vi "configure operation.vi"(7 "owner ID":refnum<class "Profibus Module configuration.lvclass">, 8 "error in":errorcluster, 10 "line item in":T1, 11 "engine configuration in":refnum<class "engine configuration.lvclass">) -> (0 "error out":errorcluster, 1 "success":bool, 2 "line item out":T1, 5 "changed":bool)   [LabVIEW 2013, in "Profibus Module editor node.lvclass"]
uses:
  Profibus Module editor node.lvclass
  permissions.ctl
  table line.ctl
  channel/Profibus channel.lvclass
  <vilib>/NI/Module Execution Interface/Engine Configuration/engine configuration.lvclass
  configuration/Profibus Module configuration.lvclass
  <vilib>/NI/Configuration Framework/serializable configuration/NISE_CEF_serializable configuration.lvclass/NISE_CEF_serializable configuration.ctl
  <vilib>/NI/Configuration Framework/serializable configuration/NISE_CEF_serializable configuration.lvclass
  <vilib>/NI/Tag Bus Module Framework/channel/TBM channel.lvclass/TBM channel.ctl
  <vilib>/NI/Tag Bus/tag/tag descriptor.lvclass/tag descriptor.ctl
  channel/Profibus channel.lvclass/Profibus channel.ctl
  <vilib>/NI/Tag Bus/tag/Data Type.ctl
  <vilib>/NI/Configuration Framework/serializable configuration/Read UID.vi
  <vilib>/NI/Tag Bus Module Framework/channel/Read channel classification.vi
  <vilib>/NI/Tag Bus/tag/read data type.vi
  channel/Read slave.vi
  channel/Read byte.vi
  channel/Read bit.vi
  <vilib>/NI/Tag Bus/tag/write tag name.vi
  <vilib>/NI/Tag Bus/tag/write data type.vi
  <vilib>/NI/Tag Bus Module Framework/channel/Write channel classification.vi
  channel/Write slave.vi
  channel/Write byte.vi
  channel/Write bit.vi
  <vilib>/NI/Tag Bus/tag/tag descriptor.lvclass
panel:
  in  "Linked Tag":i32(listbox)
  in  "Type":i32(listbox)
  in  "bit":i32
  in  "byte":i32
  in  "slave":i8
  in  "Channel Name":string
  in  "cancel":bool
  in  "ok":bool
  in  "Access Type":T2
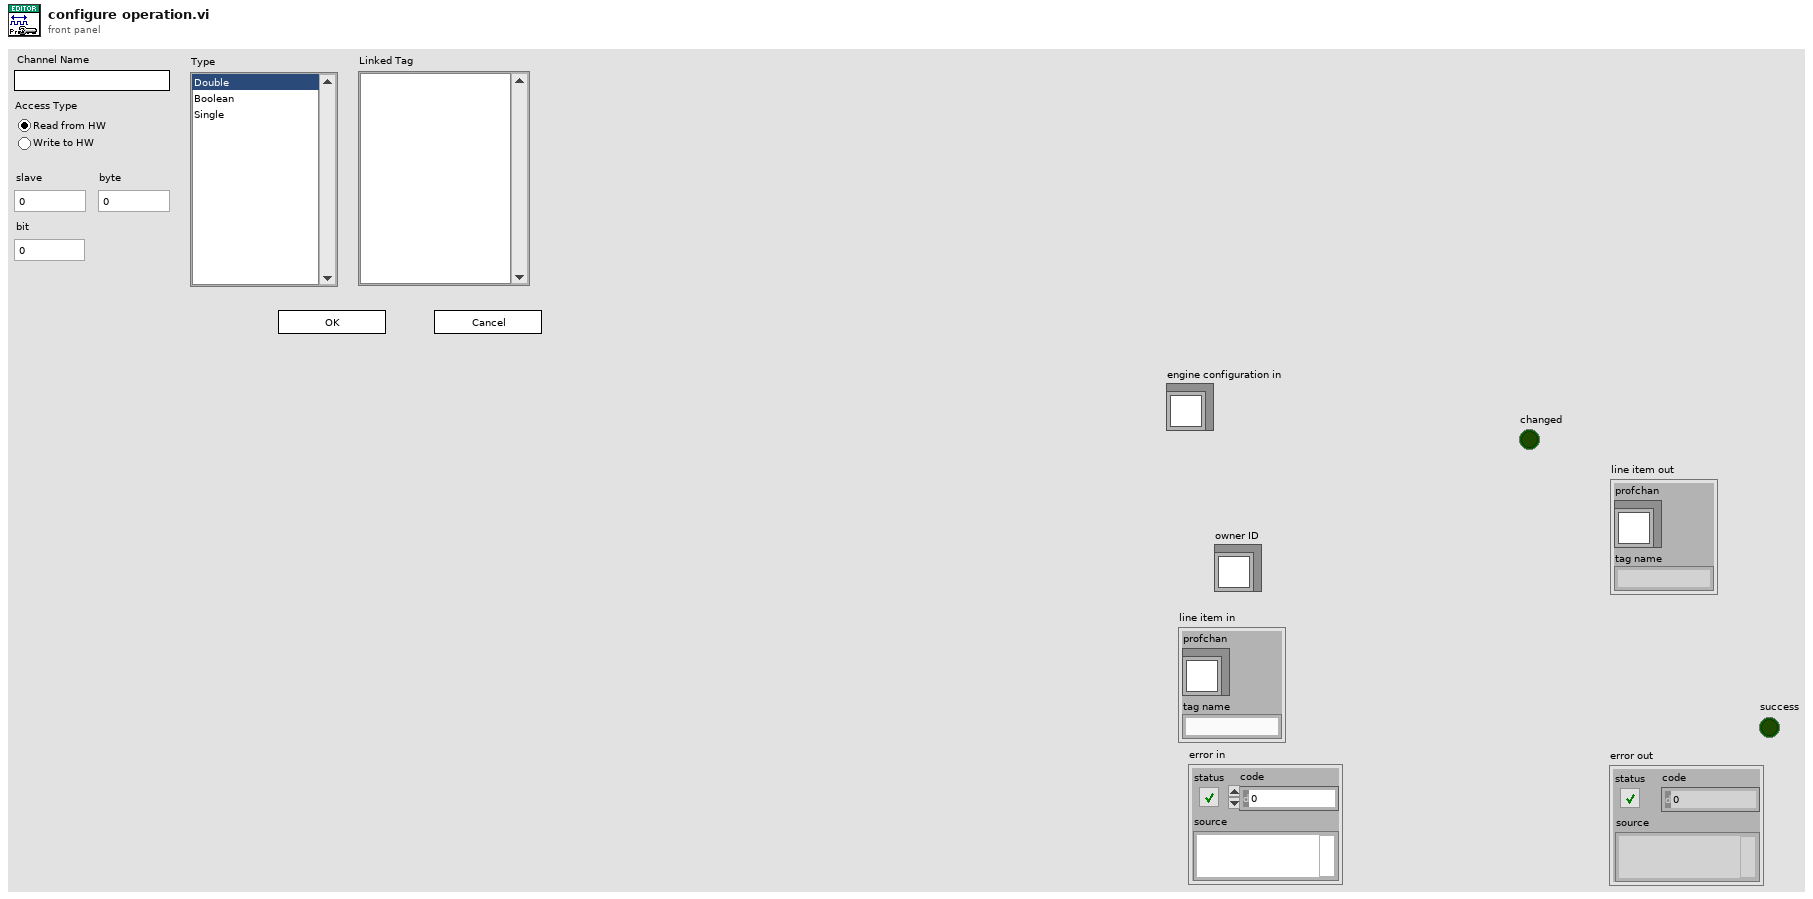
[diagram p1: front panel]
types:
  T1 = typedef "Profibus Module editor node.lvclass/table line.ctl" = cluster{"profchan":refnum<class "Profibus channel.lvclass">, "tag name":string}
  T2 = typedef "Profibus Module editor node.lvclass/permissions.ctl" = enum32{"Read from HW", "Write to HW"}
  T3 = enum32{"Invalid", "Standard", "Closed", "Hidden", "Minimized", "Maximized"}
  T4 = enum32{"Invalid", "Default", "Floating", "Floating/Auto-Hide", "Modal"}
  T5 = enum8{"Enabled", "Disabled", "Disabled and Grayed Out"}
  T6 = typedef "tag bus.lvlib/tag descriptor.lvclass/Data Type.ctl" = enum16{"Double", "Single", "I64", "I32", "I16", "I8", "U64", "U32", "U16", "U8", "Boolean", "String", "Array of Double", "Array of Single", "Array of I64", "Array of I32", "Array of I16", "Array of I8", "Array of U64", "Array of U32", "Array of U16", "Array of U8", "Array of Boolean", "Array of String"}
  T7 = enum32{"invalid app kind", "Development System", "Run Time System", "Student Edition", "Embedded LabVIEW", "Evaluation", "Custom"}
  T8 = typedef "TBM channel.lvclass/channel classification.ctl" = enum16{"input data", "output data", "processing parameter", "processing result"}
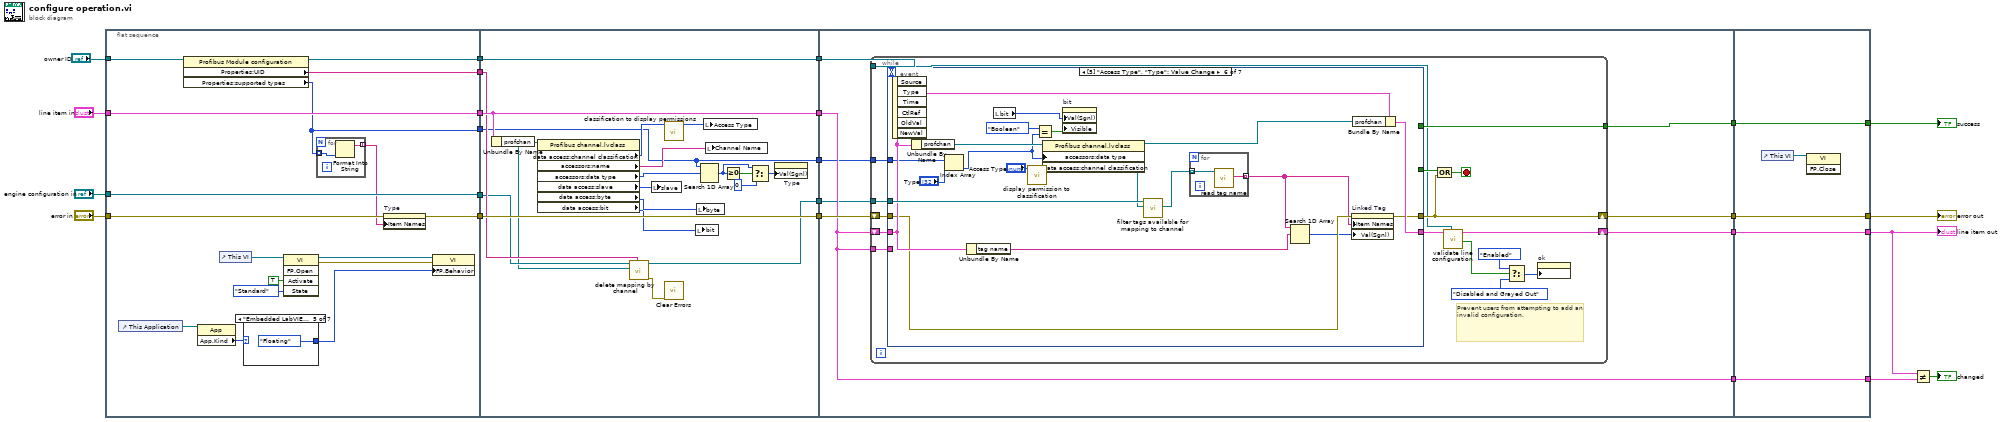
[diagram p0: block diagram]
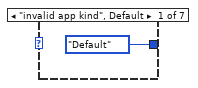
[diagram p2: hidden frame]
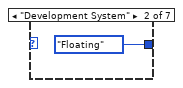
[diagram p3: hidden frame]
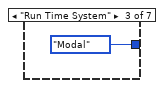
[diagram p4: hidden frame]
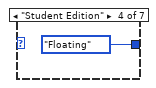
[diagram p5: hidden frame]
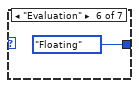
[diagram p6: hidden frame]
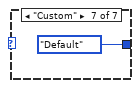
[diagram p7: hidden frame]
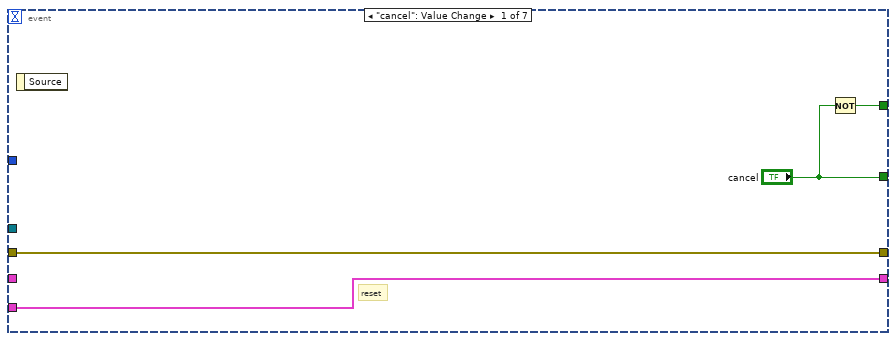
[diagram p8: hidden frame]
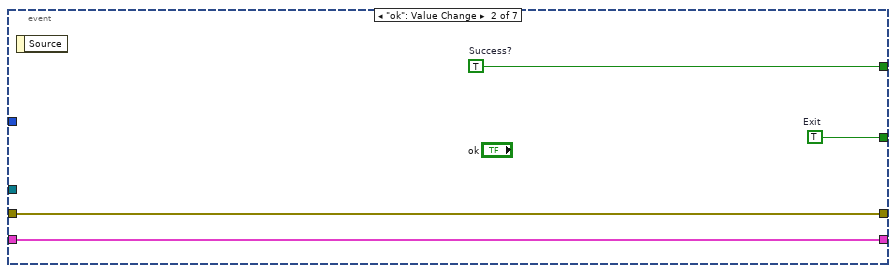
[diagram p9: hidden frame]
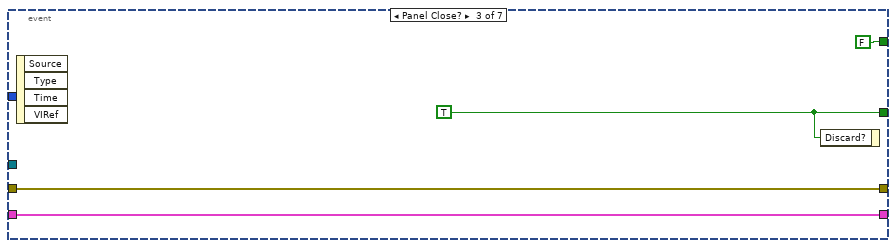
[diagram p10: hidden frame]
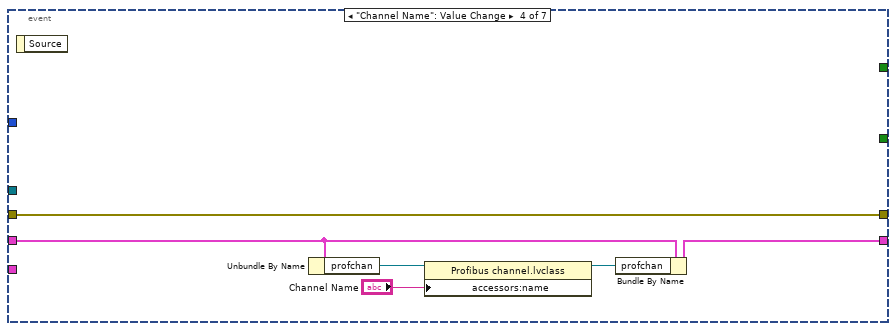
[diagram p11: hidden frame]
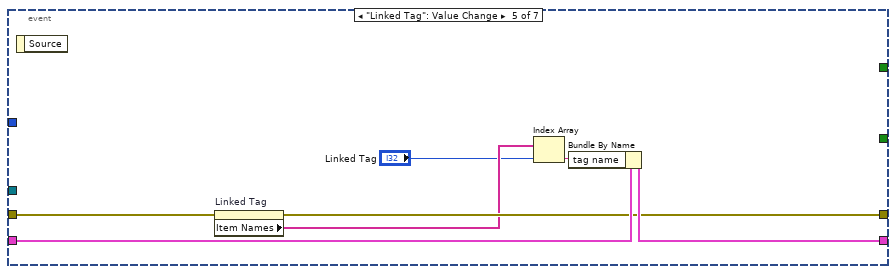
[diagram p12: hidden frame]
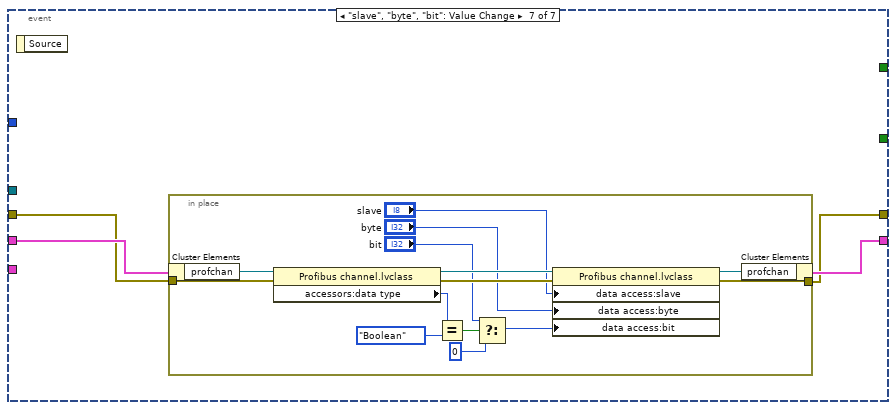
[diagram p13: hidden frame]
diagram:
  n1 = flat-sequence {
    tunnel: "line item in" -> [w41]
    tunnel: "error in" -> [w28]
    tunnel: [w27] -> w13
    tunnel: [w41] -> w11
    tunnel: [w30] -> w8
    tunnel: "owner ID" -> [w32]
    tunnel: [w31] -> w6
    tunnel: "engine configuration in" -> [w31]
    tunnel: [w29] -> w3
    tunnel: [w25] -> w2
    tunnel: w13 -> [w70]
    tunnel: [w70] -> w12
    tunnel: w11 -> [w66]
    tunnel: [w66] -> w10
    tunnel: [w62] -> w9
    tunnel: w8 -> [w62]
    tunnel: w6 -> [w59]
    tunnel: [w61] -> w4
    tunnel: w3 -> [w60]
    tunnel: w2 -> [w52]
    tunnel: [w52] -> w1
    tunnel: [w77] -> w17
    tunnel: [w76] -> w16
    tunnel: [w75] -> w15
    tunnel: [w74] -> w14
    tunnel: w12 -> [w78]
    tunnel: w10 -> [w74]
    tunnel: w9 -> [w73]
    tunnel: w4 -> [w72]
    tunnel: w1 -> [w71]
    tunnel: [w160] -> w18
    tunnel: [w161] -> w21
    tunnel: [w162] -> w22
    tunnel: [w163] -> w23
    tunnel: w17 -> [w163]
    tunnel: w16 -> [w162]
    tunnel: w15 -> [w161]
    tunnel: w14 -> [w160]
    frame #0 {
      n2 = control-ref of="This Application"() -> (w35:refnum<vi>)
      n3 = property class="Profibus Module configuration"(reference=w32) -> (reference out=w30:refnum<class "Profibus Module configuration.lvclass">, "Properties:UID"=w29:string, "Properties:supported types"=w25:T6[])  [unwired: 1 in, 1 out]
      n4 = property class="App"(reference=w35) -> ("App.Kind"=w34:T7)  [unwired: 1 in, 2 out]
      n5 = control-ref of="This VI"() -> (w36:refnum<vi>)
      n6 = case shown="\"Embedded LabVIEW\"" w34 {
        tunnel: [T4."Default" ("Front Panel Window:Behavior") T4."Floating" ("Front Panel Window:Behavior") T4."Modal" ("Front Panel Window:Behavior") T4."Floating" ("Front Panel Window:Behavior") T4."Floating" ("Front Panel Window:Behavior") T4."Floating" ("Front Panel Window:Behavior") T4."Default" ("Front Panel Window:Behavior")] -> w33
        frame "invalid app kind", Default {
        }
        frame "Development System" {
        }
        frame "Run Time System" {
        }
        frame "Student Edition" {
        }
        frame "Embedded LabVIEW" {
        }
        frame "Evaluation" {
        }
        frame "Custom" {
        }
      }
      n7 = invoke class="VI" method="FP.Open"(reference=w36, "Activate"=TRUE ("Activate?"), "State"=T3."Standard") -> (reference out=w39:refnum<vi>, error out=w40:errorcluster)  [unwired: 2 in, 3 out]
      n8 = for {
        tunnel: w25 -> [w43] mode=indexing
        tunnel: [w42] -> w26 mode=indexing
        n9 = Format Into String(w43) -> (resulting string=w42:string)  [unwired: 3 in, 1 out]
      }
      n10 = property on="Type" class="LstBox (strict)"(error in=w28, "Item Names"=w26) -> (error out=w27:errorcluster)  [unwired: 1 in, 1 out]
      n11 = property class="VI"(reference=w39, error in=w40, "FP.Behavior"=w33) -> ()  [unwired: 2 out]
    }
    frame #1 {
      n12 = Unbundle By Name(w66) -> ("profchan"=w58:refnum<class "Profibus channel.lvclass">)
      n13 = property class="Profibus channel.lvclass"(reference=w58) -> ("data access:channel classification"=w69:T8, "accessors:name"=w68:string, "accessors:data type"=w56:T6, "data access:slave"=w63:i8, "data access:byte"=w65:i32, "data access:bit"=w64:i32)  [unwired: 1 in, 2 out]
      n14 = call <vilib>:"delete mapping by channel.vi"("owner ID"=w60, "channel"=w58, "engine configuration in"=w59) -> ("error out"=w57:errorcluster, "engine configuration out"=w61:refnum<class "engine configuration.lvclass">)  [unwired: 7 in]
      n15 = local write "slave"(w63) -> ()
      n16 = call "classification to display permissions.vi"("channel classification"=w69) -> ("permissions"=w67:T2)  [unwired: 10 in]
      n17 = call <vilib>:"Clear Errors.vi"("error in (no error)"=w57) -> ()  [unwired: 6 in, 1 out]
      n18 = local write "bit"(w64) -> ()
      n19 = local write "byte"(w65) -> ()
      n20 = Search 1D Array(1D array=w52, element=w56) -> (index of element=w54:i32)  [unwired: 1 in]
      n21 = local write "Access Type"(w67) -> ()
      n22 = local write "Channel Name"(w68) -> ()
      n23 = Greater Or Equal To 0?(x=w54) -> (x >= 0?=w55:bool)
      n24 = Select(t=w54, s=w55, f=0) -> (s? t:f=w51:i32)
      n25 = property on="Type" class="LstBox (strict)"("Val(Sgnl)"=w51) -> ()  [unwired: 2 in, 2 out]
    }
    frame #2 {
      n26 = while {
        shift-right: [w86] -> w76
        shift-left: w78 -> [w81]
        tunnel: [w93] -> w77
        shift-right: [w87] -> w75
        shift-left: w74 -> [w90]
        tunnel: w74 -> [w89]
        tunnel: w73 -> [w80]
        tunnel: w71 -> [w79]
        tunnel: w72 -> [w94]
        stop <- w91 stop-if-true
        # "Prevent users from attempting to add an invalid configuration."
        n27 = event shown="[5] \"Access Type\", \"Type\": Value Change" {
          selector: _ -> [_ _ _ _ _ _ _]
          dyn-events: _ -> [_ _ _ _ _ _ _]
          timeout: _ -> [_ _ _ _ _ _ _]
          tunnel: w94 -> [_ _ _ _ _ w136 _]
          tunnel: w81 -> [w98 w102 w106 w112 w116 w123 w141]
          tunnel: [w98 w102 w106 w112 w115 w124 w142] -> w86
          tunnel: [w97 w99 FALSE _ _ _ _] -> w93
          tunnel: ["cancel" w100 w104 _ _ _ _] -> w92
          tunnel: w90 -> [_ w101 w103 w110 w119 w134 w144]
          tunnel: [w95 w101 w103 w111 w118 w128 w143] -> w88
          tunnel: w89 -> [w95 _ _ _ _ _ _]
          tunnel: w79 -> [_ _ _ _ _ w127 _]
          event "cancel": Value Change {
            # "reset"
            n28 = event-data() -> ()  [unwired: 1 in, 1 out]
            n29 = Not(x="cancel") -> (.not. x?=w97:bool)
          }
          event "ok": Value Change {
            w99 = TRUE  # Success?
            w100 = TRUE  # Exit
            n30 = event-data() -> ()  [unwired: 1 in, 1 out]
          }
          event Panel Close? {
            w104 = TRUE ("cancel")
            n31 = event-data() -> ()  [unwired: 1 in, 4 out]
            n32 = event-data("Discard?"=w104) -> ()  [unwired: 1 in, 1 out]
          }
          event "Channel Name": Value Change {
            n33 = event-data() -> ()  [unwired: 1 in, 1 out]
            n34 = Unbundle By Name(w110) -> ("profchan"=w109:refnum<class "Profibus channel.lvclass">)
            n35 = property class="Profibus channel.lvclass"(reference=w109, "accessors:name"="Channel Name") -> (reference out=w108:refnum<class "Profibus channel.lvclass">)  [unwired: 1 in, 1 out]
            n36 = Bundle By Name(cluster=w110, "profchan"=w108) -> (w111:T1)
          }
          event "Linked Tag": Value Change {
            n37 = event-data() -> ()  [unwired: 1 in, 1 out]
            n38 = property on="Linked Tag" class="LstBox (strict)"(error in=w116) -> (error out=w115:errorcluster, "Item Names"=w114:string[])  [unwired: 1 in, 1 out]
            n39 = Index Array(array=w114, index="Linked Tag") -> (element=w117:string)
            n40 = Bundle By Name(cluster=w119, "tag name"=w117) -> (w118:T1)
          }
          event "Type": Value Change {
            n41 = event-data() -> ()  [unwired: 1 in, 6 out]
            n42 = Unbundle By Name(w134) -> ("profchan"=w129:refnum<class "Profibus channel.lvclass">)
            n43 = Index Array(array=w127, index="Type") -> (element=w125:T6)
            n44 = Unbundle By Name(w134) -> ("tag name"=w121:string)
            n45 = local read "bit"() -> (w130:i32)
            n46 = call "display permission to classification.vi"("display permissions"="Access Type") -> ("channel classification"=w137:T8)  [unwired: 10 in]
            n47 = Equal?(x=Data_Type."Boolean", y=w125) -> (x = y?=w131:bool)
            n48 = property class="Profibus channel.lvclass"(reference=w129, "accessors:data type"=w125, "data access:channel classification"=w137) -> (reference out=w135:refnum<class "Profibus channel.lvclass">)  [unwired: 1 in, 1 out]
            n49 = property on="bit" class="DigNum (strict)"("Val(Sgnl)"=w130, "Visible"=w131) -> ()  [unwired: 2 in, 2 out]
            n50 = call <vilib>:"filter tags available for mapping to channel.vi"("channel to map to"=w135, "engine configuration in"=w136) -> ("filtered tags"=w133:refnum<class "tag descriptor.lvclass">[])  [unwired: 8 in, 1 out]
            n51 = for {
              tunnel: w133 -> [w140] mode=indexing
              tunnel: [w139] -> w122 mode=indexing
              n52 = call <vilib>:"read tag name.vi"("system tag in"=w140) -> ("name"=w139:string)  [unwired: 8 in, 2 out]
            }
            n53 = Search 1D Array(1D array=w122, element=w121) -> (index of element=w120:i32)  [unwired: 1 in]
            n54 = property on="Linked Tag" class="LstBox (strict)"(error in=w123, "Item Names"=w122, "Val(Sgnl)"=w120) -> (error out=w124:errorcluster)  [unwired: 1 in, 1 out]
            n55 = Bundle By Name(cluster=w134, "profchan"=w135) -> (w128:T1)
          }
          event "slave", "byte", "bit": Value Change {
            n56 = event-data() -> ()  [unwired: 1 in, 1 out]
            n57 = in-place {
              in-place-border: [w154] -> w142
              in-place-border: w141 -> [w153]
              n58 = in-place-cluster #1(w144) -> ("profchan"=w158:refnum<class "Profibus channel.lvclass">)
              n59 = property class="Profibus channel.lvclass"(reference=w158, error in=w153) -> (reference out=w156:refnum<class "Profibus channel.lvclass">, error out=w155:errorcluster, "accessors:data type"=w152:T6)
              n60 = Equal?(x=w152, y=Data_Type."Boolean") -> (x = y?=w150:bool)
              n61 = Select(t="bit", s=w150, f=0) -> (s? t:f=w147:i32)
              n62 = property class="Profibus channel.lvclass"(reference=w156, error in=w155, "data access:slave"="slave", "data access:byte"="byte", "data access:bit"=w147) -> (reference out=w157:refnum<class "Profibus channel.lvclass">, error out=w154:errorcluster)
              n63 = in-place-cluster #1("profchan"=w157) -> (w143:T1)
            }
          }
        }
        n64 = Compound Arithmetic op=OR(w92, w86) -> (w91:bool)
        n65 = call "validate line configuration.vi"("Profibus Module configuration"=w80, "line in"=w88) -> ("valid?"=w85:bool, "line out"=w87:T1)  [unwired: 8 in]
        n66 = Select(t=T5."Enabled" ("Disabled"), s=w85, f=T5."Disabled and Grayed Out") -> (s? t:f=w82:T5)
        n67 = property on="ok" class="Bool"("DisabledEnum"=w82) -> ()  [unwired: 2 in, 2 out]
      }
    }
    frame #3 {
      n68 = control-ref of="This VI"() -> (w159:refnum<vi>)
      n69 = invoke class="VI" method="FP.Close"(reference=w159) -> ()  [unwired: 2 in, 3 out]
    }
  }
  n70 = Not Equal?(x=w21, y=w18) -> (x != y?=→"changed":bool)
  "error out" <- w22
  "success" <- w23
  "line item out" <- w21
